vi "pakistan.vi"() -> ()   [LabVIEW 2011]
uses:
  VisualStudio/linking/Debug/linking.dll
panel:
  out "2D Picture":picture
  in  "Path":path
  out "X^2 + Y^2":dbl
  in  "X":dbl
  in  "Y":dbl
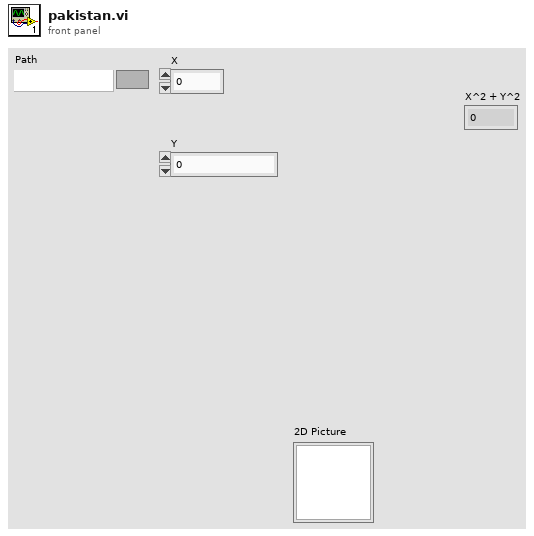
[diagram p1: front panel]
types:
  T1 = typedef "imagedata.ctl" = cluster{"image type":i32, "image depth":i32, "image":u8[], "mask":u8[], "colors":u32[], "Rectangle":cluster{"left":i16, "top":i16, "right":i16, "bottom":i16}}
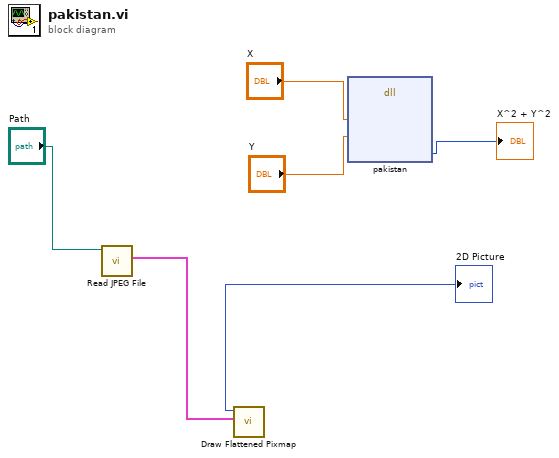
[diagram p0: block diagram]
diagram:
  n1 = call <vilib>:"Read JPEG File.vi"("path to JPEG file"="Path") -> ("image data"=w2:T1)  [unwired: 8 in, 2 out]
  n2 = call <vilib>:"Draw Flattened Pixmap.vi"("image data"=w2) -> ("new picture"=→"2D Picture":picture)  [unwired: 8 in]
  n3 = dll-call lib="C:/Users/umfehr44.ENG/Desktop/Micromirror Project/GloryofPakistanV2/VisualStudio/linking/Debug/linking.dll" fn="pakistan"("x"="X", "y"="Y") -> ("z"=→"X^2 + Y^2":i32)  [unwired: 7 in, 2 out]
